vi "CONF digital clear.vi"(8 "error in (no error)":errorcluster, 11 "Digital ref out":T1) -> (0 "error out":errorcluster)   [LabVIEW 2013]
doc: "Use this template to build a VI to use as a subVI."
uses:
  Kontrolki/KartaDAQ/CONF Digital Refnum.ctl
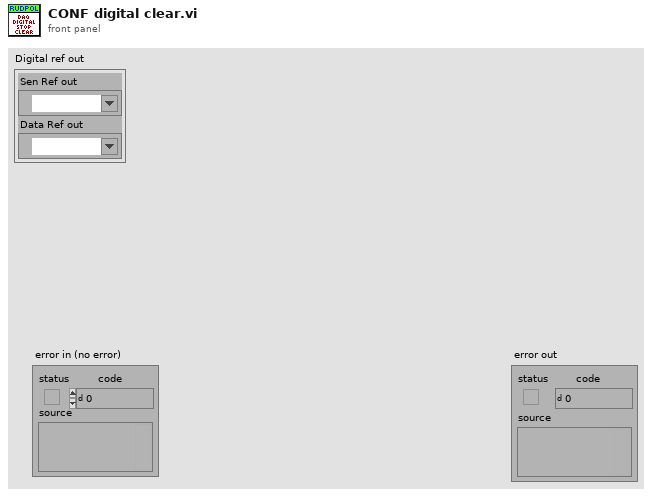
[diagram p1: front panel]
types:
  T1 = typedef "CONF Digital Refnum.ctl" = cluster{"Sen Ref out":refnum<k21>, "Data Ref out":refnum<k21>}
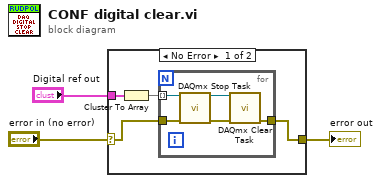
[diagram p0: block diagram]
diagram:
  n1 = case shown="No Error" "error in (no error)" {
    selector: "error in (no error)" -> [w5 w13]
    tunnel: [w4 w13] -> w2
    tunnel: "Digital ref out" -> [w7 _]
    frame No Error {
      n2 = Cluster To Array(cluster=w7) -> (array=w6:refnum<k21>[])
      n3 = for {
        tunnel: w6 -> [w10] mode=indexing
        tunnel: w5 -> [w9]
        tunnel: [w8] -> w4
        n4 = call <vilib>:"DAQmx Stop Task.vi"("task/channels in"=w10, "error in"=w9) -> ("task out"=w11:refnum<k21>, "error out"=w12:errorcluster)  [unwired: 12 in]
        n5 = call <vilib>:"DAQmx Clear Task.vi"("task in"=w11, "error in"=w12) -> ("error out"=w8:errorcluster)  [unwired: 13 in]
      }
    }
    frame Error {
    }
  }
  "error out" <- w2
